vi "Test1.vi"() -> ()   [LabVIEW 2014]
panel:
  out "Meter":dbl(knob) scale=0.0..10.0
  in  "Boolean":bool
  in  "Numeric 2":dbl
  in  "Numeric":dbl
  # "Adds the two numbers if Boolean is true, otherwise displays only the first value."
  # "You could add something simple for testing"
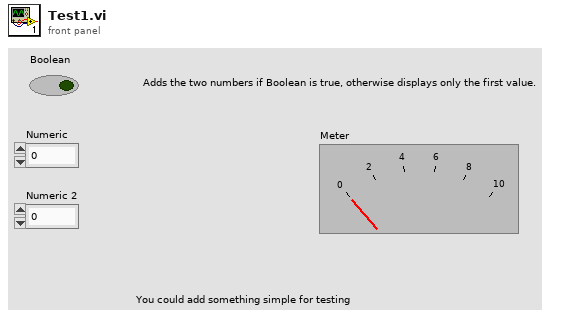
[diagram p1: front panel]
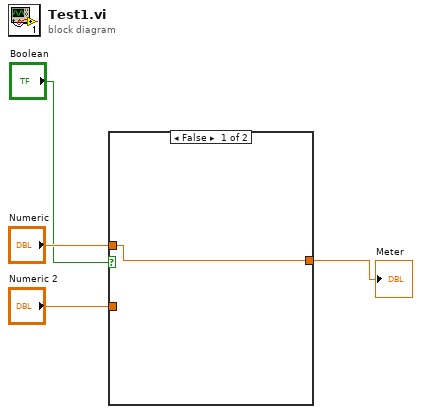
[diagram p0: block diagram]
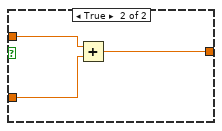
[diagram p2: hidden frame]
diagram:
  n1 = case shown="False" "Boolean" {
    tunnel: "Numeric" -> [w5 w8]
    tunnel: "Numeric 2" -> [_ w7]
    tunnel: [w5 w6] -> w2
    frame False {
    }
    frame True {
      n2 = Add(x=w8, y=w7) -> (x+y=w6:dbl)
    }
  }
  "Meter" <- w2
